vi "open connection.vi"(8 "error in (no error)":errorcluster caption="Fehler (Eingang, kein Fehler)", 11 "DeviceInterface Eingang":refnum<class "DeviceInterface.lvclass"> caption="DNL_LabVIEW Object in") -> (0 "error out":errorcluster caption="Fehler (Ausgang)", 3 "DeviceInterface Ausgang":refnum<class "DeviceInterface.lvclass"> caption="DNL_LabVIEW Object out")   [LabVIEW 2013, in "DeviceInterface.lvclass"]
doc: "Verbindung zu dem Gerät öffnen"
uses:
  DeviceInterface.lvclass
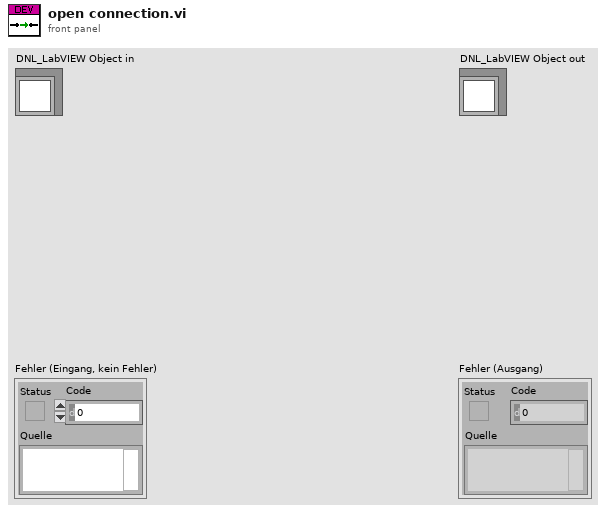
[diagram p1: front panel]
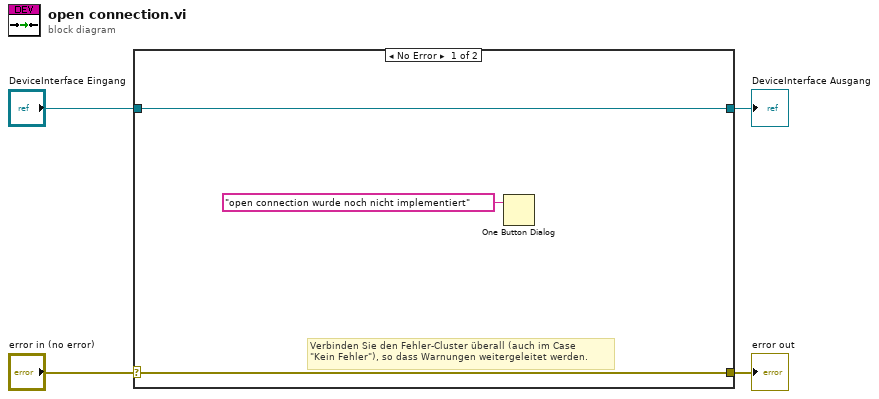
[diagram p0: block diagram]
diagram:
  n1 = case shown="No Error" "error in (no error)" {
    selector: "error in (no error)" -> [w6 w9]
    tunnel: [w6 w9] -> w3
    tunnel: [w7 w8] -> w1
    tunnel: "DeviceInterface Eingang" -> [w7 w8]
    frame No Error {
      # "Verbinden Sie den Fehler-Cluster überall (auch im Case\n\"Kein Fehler\"), so dass Warnungen weitergeleitet werden."
      n2 = One Button Dialog(message="open connection wurde noch nicht implementiert" ("Nachricht")) -> ()  [unwired: 1 in, 1 out]
    }
    frame Error {
    }
  }
  "error out" <- w3
  "DeviceInterface Ausgang" <- w1
